vi "Configure Trigger.vi"(8 "error in":errorcluster, 10 "Trigger Type":T1(ring), 11 "FPGA VI Reference In":refnum<k20>) -> (0 "error out":errorcluster, 3 "FPGA VI Reference Out":refnum<k20>)   [LabVIEW 2012]
uses:
  <vilib>/Utility/error.llb/Error Cluster From Error Code.vi
  <vilib>/rvi/errors/niLvFpgaAdjustHostInterfaceError.vi
  <vilib>/rvi/interface/nirviReadWriteControl/nirviReadWriteControl.xnode
  NiFpgaLv.dll
  <vilib>/rvi/interface/Simulation/niFpgaSimulationCallBeginRW.vi
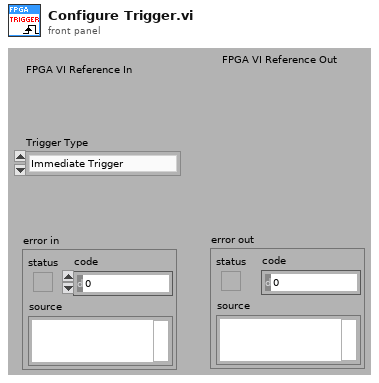
[diagram p1: front panel]
types:
  T1 = enum8{"Immediate Trigger", "Software Trigger", "External Digital Trigger", "Analog Trigger"}
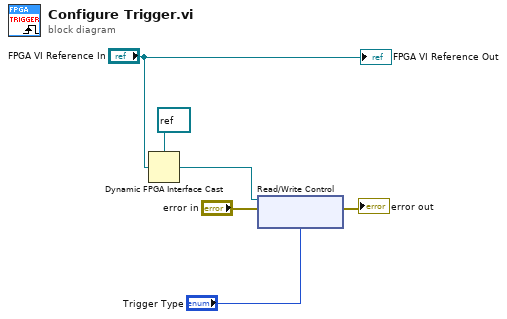
[diagram p0: block diagram]
diagram:
  n1 = Dynamic FPGA Interface Cast(Session In=refnum<k20> refnum ("Type"), Type="FPGA VI Reference In") -> (Session Out=w3:refnum<k20>)
  n2 = xnode "Read/Write Control"("FPGA VI Reference In"=w3, "error in"="error in", "Trigger Type"="Trigger Type") -> ("error out"=→"error out":errorcluster)  [unwired: 1 out]
  "FPGA VI Reference Out" <- "FPGA VI Reference In"
